vi "readModbus.vi"(8 "error in (no error)":errorcluster, 10 "E_values":T1, 11 "VISA resource name":refnum<visa-resource-name>) -> (0 "error out":errorcluster, 2 "E_values 2":T1, 3 "VISA Refnum out":refnum<visa-resource-name>)   [LabVIEW 2026]
panel:
  out "E_muneca":u32(knob) scale=0.0..400.0
  out "E_antebrazo":u32(knob) scale=0.0..400.0
  out "E_codo":u32(knob) scale=0.0..400.0
  out "E_hombro":u32(knob) scale=0.0..400.0
  out "E_cadera":u32(knob) scale=0.0..400.0
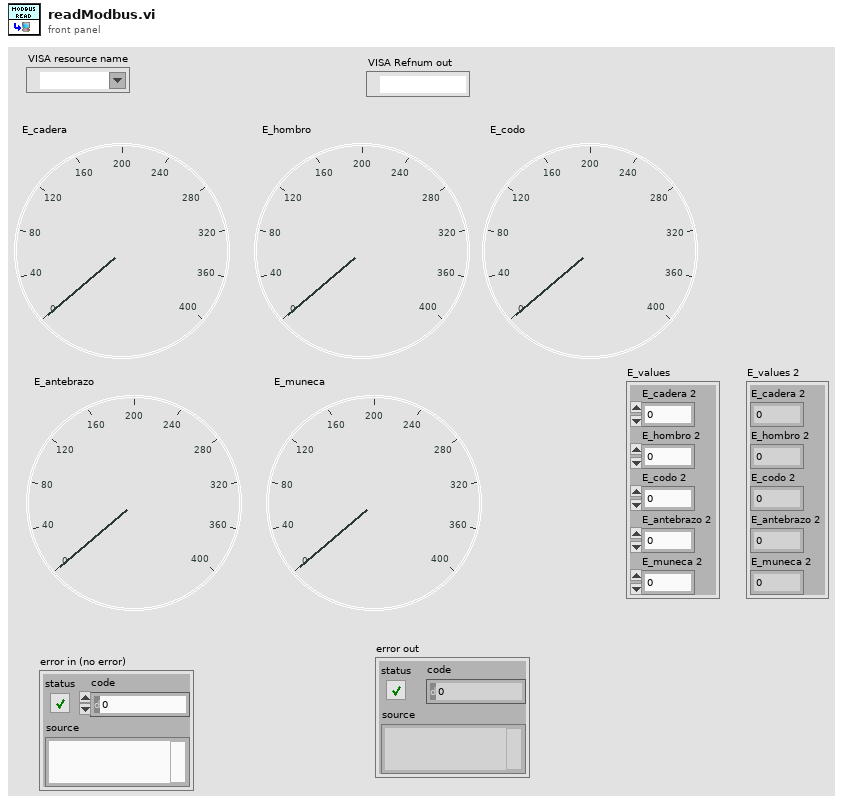
[diagram p1: front panel]
types:
  T1 = cluster{"E_cadera 2":u32, "E_hombro 2":u32, "E_codo 2":u32, "E_antebrazo 2":u32, "E_muneca 2":u32}
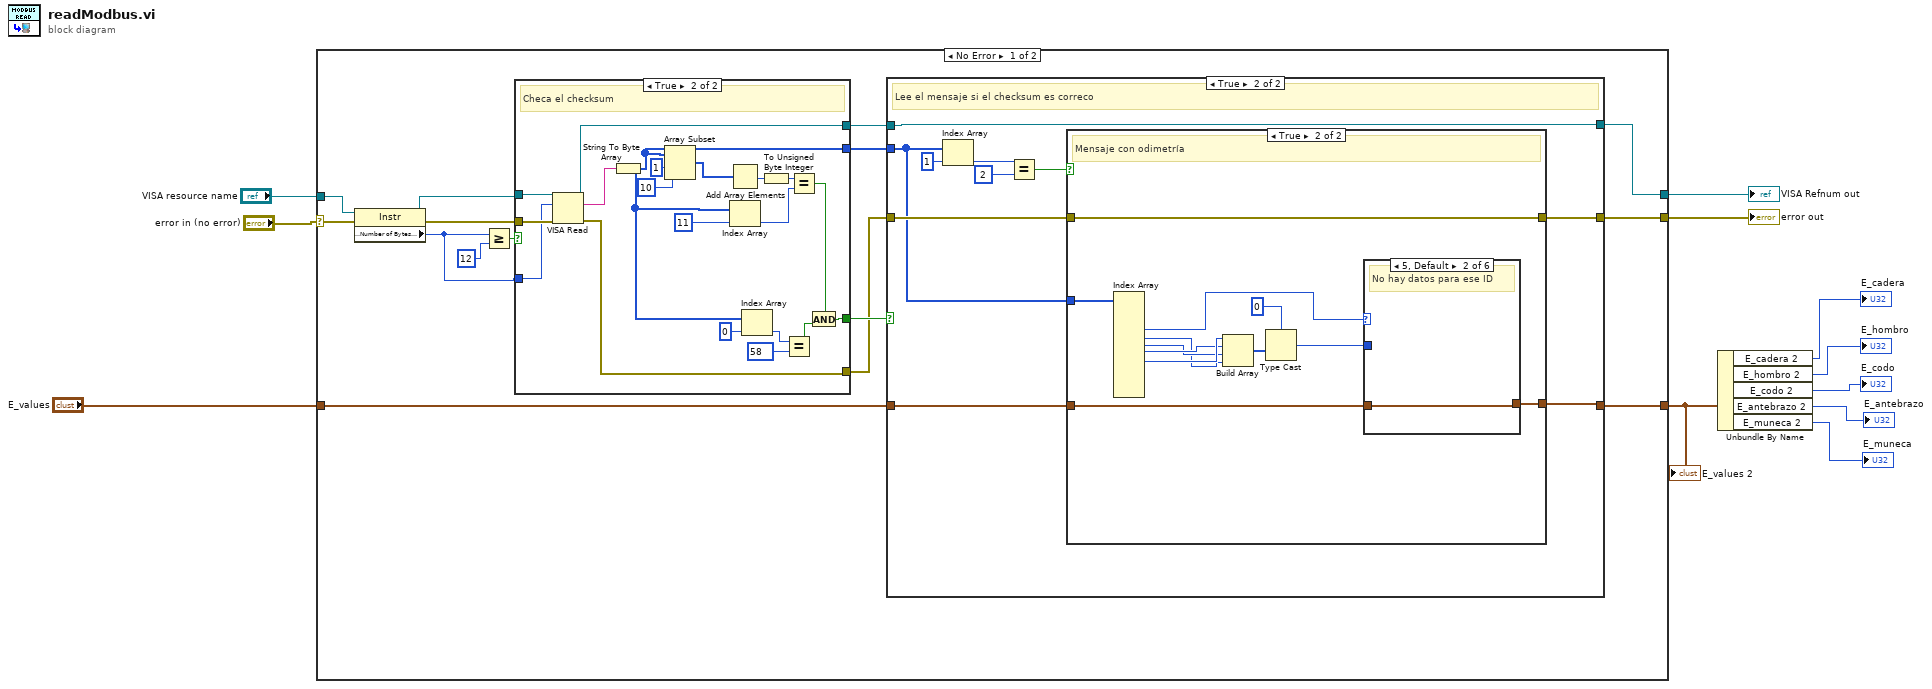
[diagram p0: block diagram]
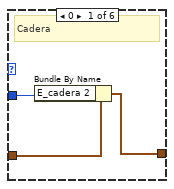
[diagram p4: hidden frame]
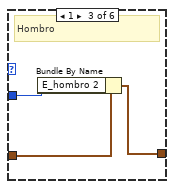
[diagram p5: hidden frame]
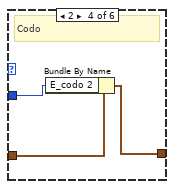
[diagram p6: hidden frame]
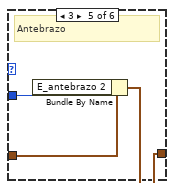
[diagram p7: hidden frame]
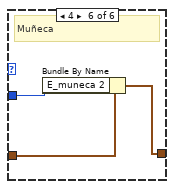
[diagram p8: hidden frame]
diagram:
  n1 = case shown="No Error" "error in (no error)" {
    selector: "error in (no error)" -> [w25 w94]
    tunnel: "VISA resource name" -> [w26 w95]
    tunnel: [w15 w94] -> w9
    tunnel: [w17 w95] -> w8
    tunnel: "E_values" -> [w13 w93]
    tunnel: [w12 w93] -> w7
    frame No Error {
      n2 = property class="Instr"(reference=w26, error in=w25) -> (reference out=w21:refnum<visa-resource-name>, error out=w22:errorcluster, "Serial Settings:Number of Bytes at Serial Port"=w20:u32)
      n3 = Greater Or Equal?(x=w20, y=u32 12) -> (x >= y?=w23:bool)
      n4 = case shown="True" w23 {
        selector: w23 -> [w70 _]
        tunnel: w22 -> [w72 w92]
        tunnel: w21 -> [w71 w91]
        tunnel: w20 -> [_ w90]
        tunnel: [w72 w82] -> w16
        tunnel: [w71 w83] -> w18
        tunnel: [w70 w81] -> w19
        tunnel: [_ w73] -> w14
        frame False {
          # "Mensaje incompleto (menos de 12 bytes)"
        }
        frame True {
          # "Checa el checksum"
          n5 = VISA Read(VISA resource name=w91, byte count=w90, error in (no error)=w92) -> (VISA resource name out=w83:refnum<visa-resource-name>, read buffer=w89:string, error out=w82:errorcluster)  [unwired: 1 out]
          n6 = String To Byte Array(string=w89) -> (unsigned byte array=w73:u8[])
          n7 = Array Subset(array=w73, index=1, length=10) -> (w78:u8[])
          n8 = Add Array Elements(numeric array=w78) -> (sum=w88:u8)
          n9 = Index Array(array=w73, index=11) -> (element=w85:u8)
          n10 = Index Array(array=w73, index=0) -> (element=w74:u8)
          n11 = To Unsigned Byte Integer(number=w88) -> (unsigned 8bit integer=w75:u8)
          n12 = Equal?(x=w74, y=u8 58) -> (x = y?=w76:bool)
          n13 = Equal?(x=w75, y=w85) -> (x = y?=w80:bool)
          n14 = And(x=w80, y=w76) -> (x .and. y?=w81:bool)
        }
      }
      n15 = case shown="True" w19 {
        tunnel: w18 -> [w29 w31]
        tunnel: [w29 w31] -> w17
        tunnel: w16 -> [w28 w33]
        tunnel: [w28 w32] -> w15
        tunnel: w14 -> [_ w30]
        tunnel: w13 -> [w27 w35]
        tunnel: [w27 w34] -> w12
        frame False {
        }
        frame True {
          # "Lee el mensaje si el checksum es correco"
          n16 = Index Array(array=w30, index=1) -> (element=w37:u8)
          n17 = Equal?(x=w37, y=u8 2) -> (x = y?=w36:bool)
          n18 = case shown="True" w36 {
            tunnel: [w41 w51] -> w34
            tunnel: w35 -> [w41 w48]
            tunnel: w33 -> [w40 w50]
            tunnel: [w40 w50] -> w32
            tunnel: w30 -> [_ w49]
            frame False {
              # "Se mantienen los valores (el mensaje es incorrecto)"
            }
            frame True {
              # "Mensaje con odimetría"
              n19 = Index Array(array=w49) -> (element #3=w47:u8, element #4=w42:u8, element #5=w43:u8, element #6=w44:u8, element #7=w45:u8)  [unwired: 11 in, 6 out]
              n20 = Build Array(w45, w44, w43, w42) -> (w53:u8[])
              n21 = Type Cast(type=u32 0, x=w53) -> (*(type *) &x=w52:u32)
              n22 = case shown="5, Default" w47 {
                tunnel: [w56 w57 w60 w62 w65 w68] -> w51
                tunnel: w52 -> [w55 _ w59 w63 w66 w69]
                tunnel: w48 -> [w54 w57 w58 w61 w64 w67]
                frame 0 {
                  # "Cadera"
                  n23 = Bundle By Name(cluster=w54, "E_cadera 2"=w55) -> (w56:T1)
                }
                frame 5, Default {
                  # "No hay datos para ese ID"
                }
                frame 1 {
                  # "Hombro"
                  n24 = Bundle By Name(cluster=w58, "E_hombro 2"=w59) -> (w60:T1)
                }
                frame 2 {
                  # "Codo"
                  n25 = Bundle By Name(cluster=w61, "E_codo 2"=w63) -> (w62:T1)
                }
                frame 3 {
                  # "Antebrazo"
                  n26 = Bundle By Name(cluster=w64, "E_antebrazo 2"=w66) -> (w65:T1)
                }
                frame 4 {
                  # "Muñeca"
                  n27 = Bundle By Name(cluster=w67, "E_muneca 2"=w69) -> (w68:T1)
                }
              }
            }
          }
        }
      }
    }
    frame Error {
    }
  }
  "VISA Refnum out" <- w8
  "error out" <- w9
  "E_values 2" <- w7
  n28 = Unbundle By Name(w7) -> ("E_cadera 2"=→"E_cadera":u32, "E_hombro 2"=→"E_hombro":u32, "E_codo 2"=→"E_codo":u32, "E_antebrazo 2"=→"E_antebrazo":u32, "E_muneca 2"=→"E_muneca":u32)
